vi "simple caluculator.vi"() -> ()   [LabVIEW 2018]
panel:
  out "Numeric 6":dbl
  in  "Numeric 5":dbl
  in  "Numeric 4":dbl
  out "Numeric 3":dbl
  in  "Numeric 2":dbl
  in  "Numeric":dbl
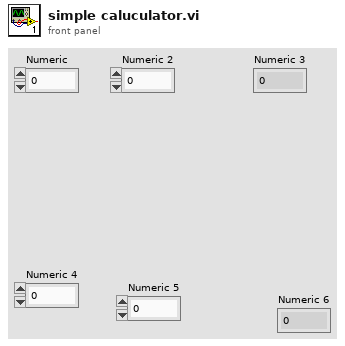
[diagram p1: front panel]
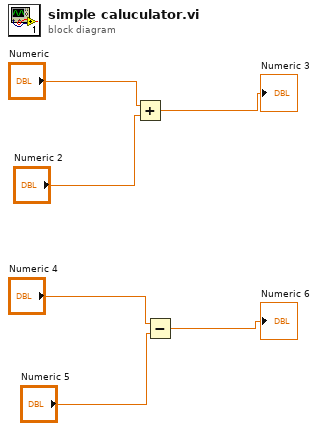
[diagram p0: block diagram]
diagram:
  n1 = Add(x="Numeric", y="Numeric 2") -> (x+y=→"Numeric 3":dbl)
  n2 = Subtract(x="Numeric 4", y="Numeric 5") -> (x-y=→"Numeric 6":dbl)
